vi "Retroparticle Area Scoring.vi"(10 "Rectangle Array ltrb":dbl[](array[numeric])=[2.22, 1.4], 11 "Particle Area":dbl) -> (3 "Score":dbl)   [LabVIEW 2015]
doc: "Calculate a score based on area and convex hull area. Convex hull area fills holes and convex areas of the shape. It is equivalent to putting a rubbed band around the shape and computing the area of the band."
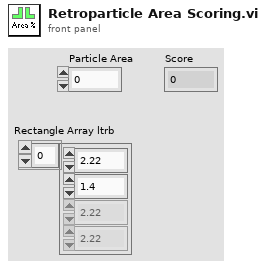
[diagram p1: front panel]
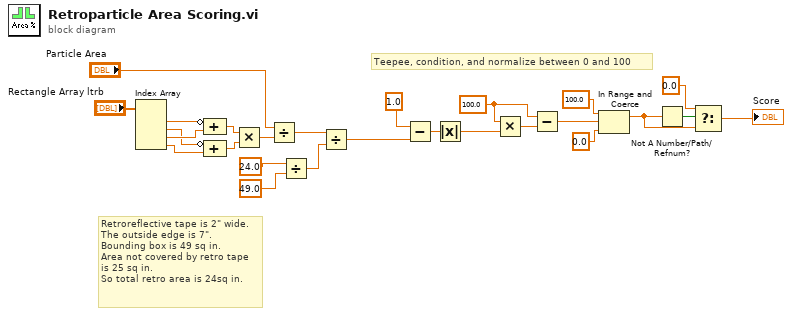
[diagram p0: block diagram]
diagram:
  w19 = 100.0 ("x/y")
  # "Retroreflective tape is 2\" wide.\nThe outside edge is 7\".\nBounding box is 49 sq in.\nArea not covered by retro tape\nis 25 sq in.\nSo total retro area is 24sq in."
  # "Teepee, condition, and normalize between 0 and 100"
  n1 = Index Array(array="Rectangle Array ltrb") -> (element #1=w11:dbl, element #2=w9:dbl, element #3=w10:dbl, element #4=w8:dbl)  [unwired: 4 in]
  n2 = Compound Arithmetic op=ADD(invert w11, w10) -> (w7:dbl)
  n3 = Compound Arithmetic op=ADD(invert w9, w8) -> (w6:dbl)
  n4 = Multiply(x=w7, y=w6) -> (x*y=w5:dbl)
  n5 = Divide(x="Particle Area", y=w5) -> (x/y=w3:dbl)
  n6 = Divide(x=24.0 ("length"), y=49.0 ("length")) -> (x/y=w2:dbl)
  n7 = Divide(x=w3, y=w2) -> (x/y=w1:dbl)
  n8 = Subtract(x=1.0 ("y"), y=w1) -> (x-y=w17:dbl)
  n9 = Absolute Value(x=w17) -> (abs(x)=w20:dbl)
  n10 = Multiply(x=w19, y=w20) -> (x*y=w21:dbl)
  n11 = Subtract(x=w19, y=w21) -> (x-y=w16:dbl)
  n12 = In Range and Coerce(upper limit=100.0, x=w16, lower limit=0.0) -> (coerced(x)=w24:dbl)  [unwired: 1 out]
  n13 = Not A Number/Path/Refnum?(number/path/refnum=w24) -> (NaN/Path/Refnum?=w23:bool)
  n14 = Select(t=0.0 ("y"), s=w23, f=w24) -> (s? t:f=→"Score":dbl)
